vi "3.3.vi"() -> ()   [LabVIEW 2017]
uses:
  <vilib>/regexp/Match Regular Expression.xnode
panel:
  out "数值":dbl
  out "匹配之后":string
  out "所有匹配":string
  out "匹配之前":string
  in  "偏移量(0)":i32
  in  "正则表达式":string
  in  "输入字符串":string
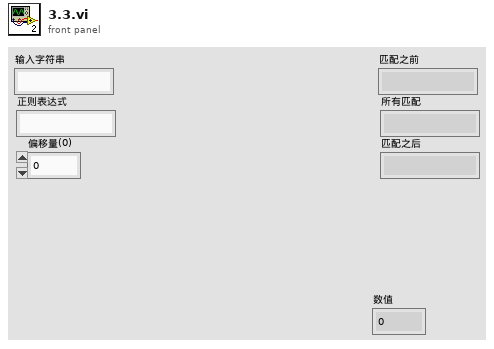
[diagram p1: front panel]
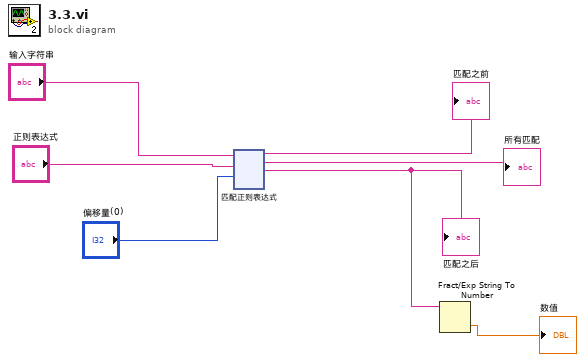
[diagram p0: block diagram]
diagram:
  n1 = xnode "匹配正则表达式"("输入字符串"="输入字符串", "正则表达式"="正则表达式", "偏移量(0)"="偏移量(0)") -> ("匹配之前"=→"匹配之前":string, "所有匹配"=→"所有匹配":string, "匹配之后"=w2:string)  [unwired: 3 in, 2 out]
  "匹配之后" <- w2
  n2 = Fract/Exp String To Number(string=w2) -> (number=→"数值":dbl)  [unwired: 3 in, 1 out]
